vi "CMD-ME stream.vi"() -> ()   [LabVIEW 2020]
uses:
  <vilib>/Instr/_visa.llb/VISA Configure Serial Port (Instr).vi
panel:
  out "String":string
  in  "baud rate (38400)":u32=9600
  in  "COM Port":refnum<visa-resource-name>
  in  "Stop":bool
  in  "Start":bool
  # "Streams data in format of              CMD-ME / Geoprospectors Version"
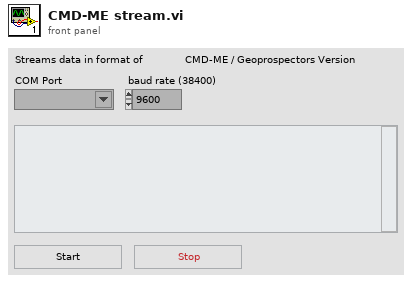
[diagram p1: front panel]
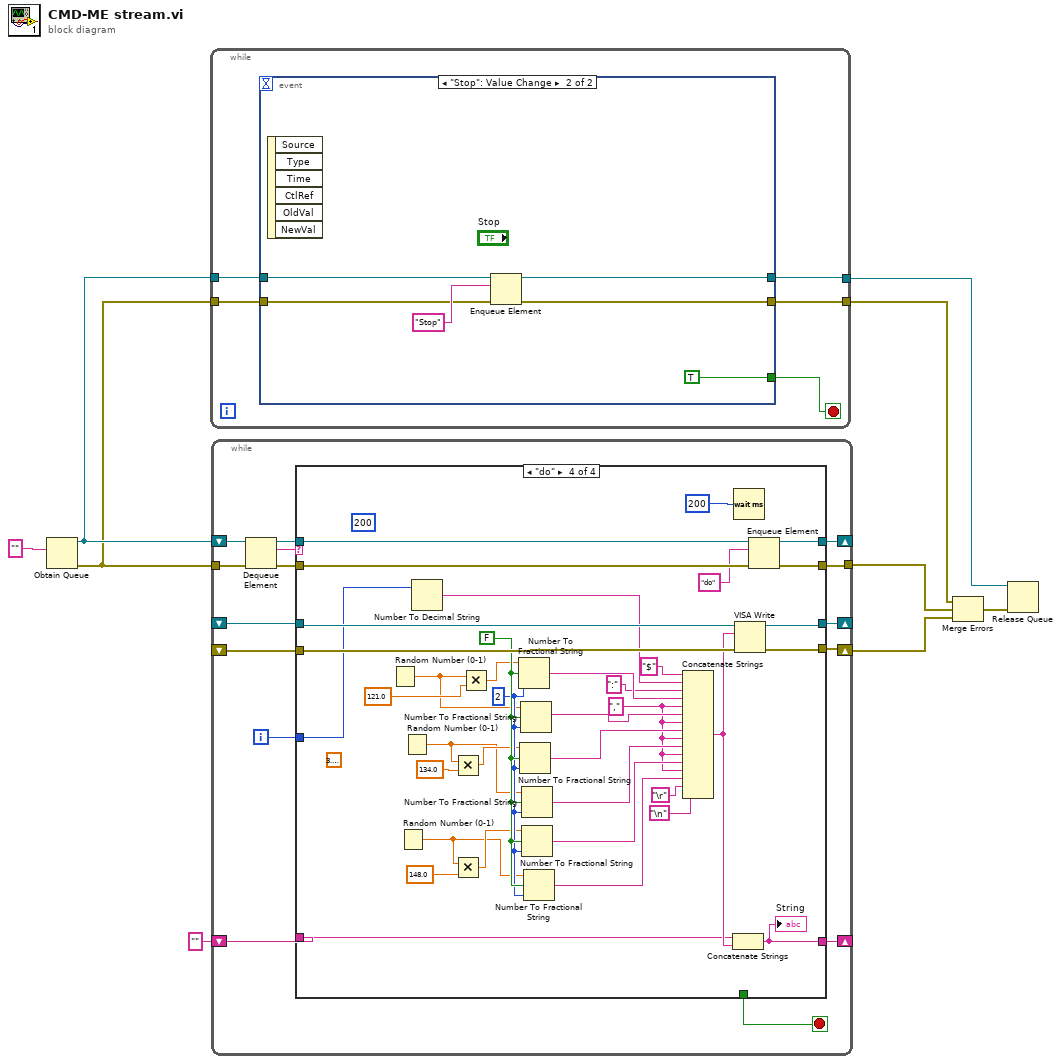
[diagram p0: block diagram]
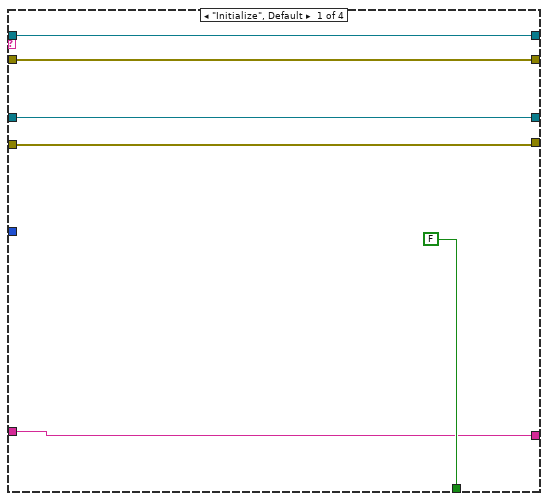
[diagram p2: hidden frame]
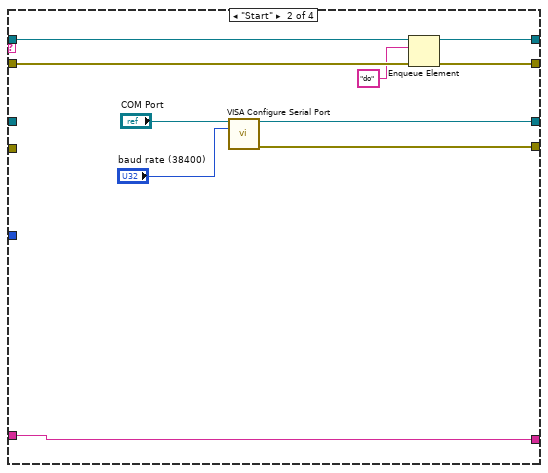
[diagram p3: hidden frame]
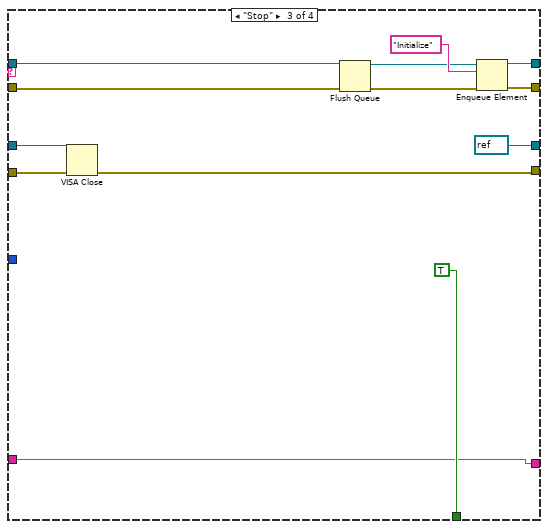
[diagram p4: hidden frame]
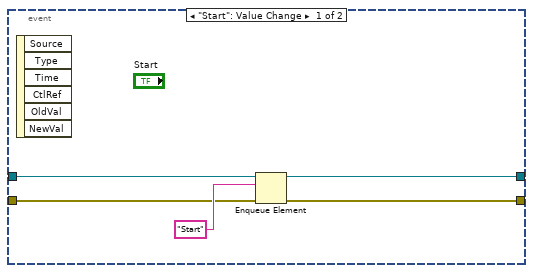
[diagram p5: hidden frame]
diagram:
  n1 = Obtain Queue(element data type="") -> (queue out=w9:refnum<queue>, error out=w7:errorcluster)  [unwired: 4 in, 1 out]
  n2 = while {
    tunnel: w9 -> [w14]
    tunnel: [w13] -> w2
    tunnel: w7 -> [w12]
    tunnel: [w11] -> w4
    stop <- w10 stop-if-true
    n3 = event shown="[1] \"Stop\": Value Change" {
      selector: _ -> [_ _]
      dyn-events: _ -> [_ _]
      timeout: _ -> [_ _]
      tunnel: w14 -> [w19 w25]
      tunnel: [w18 w23] -> w13
      tunnel: w12 -> [w16 w21]
      tunnel: [w15 w20] -> w11
      tunnel: [_ TRUE] -> w10
      event "Start": Value Change {
        n4 = event-data() -> ()  [unwired: 1 in, 6 out]
        n5 = Enqueue Element(queue=w19, element="Start", error in (no error)=w16) -> (queue out=w18:refnum<queue>, error out=w15:errorcluster)  [unwired: 1 in, 1 out]
      }
      event "Stop": Value Change {
        n6 = event-data() -> ()  [unwired: 1 in, 6 out]
        n7 = Enqueue Element(queue=w25, element="Stop", error in (no error)=w21) -> (queue out=w23:refnum<queue>, error out=w20:errorcluster)  [unwired: 1 in, 1 out]
      }
    }
  }
  n8 = while {
    shift-right: [w38] -> _
    shift-left: _ -> [w36]
    shift-right: [w37] -> w6
    shift-left: _ -> [w35]
    tunnel: [w31] -> w5
    shift-right: [w32] -> _
    shift-left: w9 -> [w40]
    tunnel: w7 -> [w30]
    shift-right: [w27] -> _
    shift-left: "" -> [w26]
    i -> [w28]
    stop <- w29 stop-if-true
    n9 = Dequeue Element(queue=w40, error in (no error)=w30) -> (queue out=w34:refnum<queue>, element=w39:string, error out=w33:errorcluster)  [unwired: 1 in, 1 out]
    n10 = case shown="\"do\"" w39 {
      tunnel: [w44 w54 refnum<visa-resource-name> refnum ("VISA resource name out") w99] -> w38
      tunnel: [w43 w53 w64 w98] -> w37
      tunnel: w36 -> [w44 _ w65 w100]
      tunnel: w35 -> [w43 _ w66 w101]
      tunnel: w34 -> [w46 w51 w58 w106]
      tunnel: w33 -> [w45 w52 w59 w105]
      tunnel: [w46 w50 w69 w104] -> w32
      tunnel: [w45 w49 w68 w103] -> w31
      tunnel: [FALSE _ TRUE _] -> w29
      tunnel: w28 -> [_ _ _ w76]
      tunnel: [w41 w47 w57 w77] -> w27
      tunnel: w26 -> [w41 w47 w57 w78]
      frame "Initialize", Default {
      }
      frame "Start" {
        n11 = call-poly "VISA Configure Serial Port"("VISA resource name"="COM Port", "baud rate (9600)"="baud rate (38400)") -> ("VISA resource name out"=w54:refnum<visa-resource-name>, "error out"=w53:errorcluster)  [unwired: 12 in]
        n12 = Enqueue Element(queue=w51, element="do", error in (no error)=w52) -> (queue out=w50:refnum<queue>, error out=w49:errorcluster)  [unwired: 1 in, 1 out]
      }
      frame "Stop" {
        n13 = VISA Close(VISA resource name=w65, error in (no error)=w66) -> (error out=w64:errorcluster)
        n14 = Flush Queue(queue=w58, error in (no error)=w59) -> (queue out=w61:refnum<queue>, error out=w60:errorcluster)  [unwired: 1 out]
        n15 = Enqueue Element(queue=w61, element="Initialize", error in (no error)=w60) -> (queue out=w69:refnum<queue>, error out=w68:errorcluster)  [unwired: 1 in, 1 out]
      }
      frame "do" {
        w92 = 2
        w86 = ","
        w94 = FALSE
        (unwired) 3.141592653589793
        (unwired) 200
        n16 = Random Number (0-1)() -> (number: 0 to 1=w74:dbl)
        n17 = Random Number (0-1)() -> (number: 0 to 1=w70:dbl)
        n18 = Random Number (0-1)() -> (number: 0 to 1=w72:dbl)
        n19 = Number To Decimal String(number=w76) -> (decimal integer string=w83:string)  [unwired: 1 in]
        n20 = Multiply(x=w72, y=134.0) -> (x*y=w73:dbl)
        n21 = Multiply(x=w70, y=148.0) -> (x*y=w71:dbl)
        n22 = Multiply(x=w74, y=121.0) -> (x*y=w75:dbl)
        n23 = Number To Fractional String(use system decimal point (T)=w94, number=w75, precision (6)=w92) -> (F-format string=w91:string)  [unwired: 1 in]
        n24 = Number To Fractional String(use system decimal point (T)=w94, number=w73, precision (6)=w92) -> (F-format string=w89:string)  [unwired: 1 in]
        n25 = Number To Fractional String(use system decimal point (T)=w94, number=w74, precision (6)=w92) -> (F-format string=w90:string)  [unwired: 1 in]
        n26 = Number To Fractional String(use system decimal point (T)=w94, number=w72, precision (6)=w92) -> (F-format string=w88:string)  [unwired: 1 in]
        n27 = Number To Fractional String(use system decimal point (T)=w94, number=w71, precision (6)=w92) -> (F-format string=w87:string)  [unwired: 1 in]
        n28 = Number To Fractional String(use system decimal point (T)=w94, number=w70, precision (6)=w92) -> (F-format string=w85:string)  [unwired: 1 in]
        n29 = Concatenate Strings("$", w83, ":", w91, w86, w90, w86, w89, w86, w88, w86, w87, w86, w85, "\r", "\n") -> (w79:string)
        n30 = Concatenate Strings(w78, w79) -> (w77:string)
        "String" <- w77
        n31 = Wait (ms)(milliseconds to wait=200) -> ()  [unwired: 1 out]
        n32 = VISA Write(VISA resource name=w100, write buffer=w79, error in (no error)=w101) -> (VISA resource name out=w99:refnum<visa-resource-name>, error out=w98:errorcluster)  [unwired: 1 out]
        n33 = Enqueue Element(queue=w106, element="do", error in (no error)=w105) -> (queue out=w104:refnum<queue>, error out=w103:errorcluster)  [unwired: 1 in, 1 out]
      }
    }
  }
  n34 = Merge Errors(w4, w5, w6) -> (w3:errorcluster)
  n35 = Release Queue(queue=w2, error in (no error)=w3) -> ()  [unwired: 1 in, 3 out]
